vi "SavedSettingsItemData.vi"(8 "error in (no error)":errorcluster, 9 "Description":string, 10 "Title":string, 11 "CtrlTree in":refnum<vi>) -> (0 "error out":errorcluster, 2 "Is Empty":bool, 3 "Data to be saved":string[](array[string]))   [LabVIEW 2021]
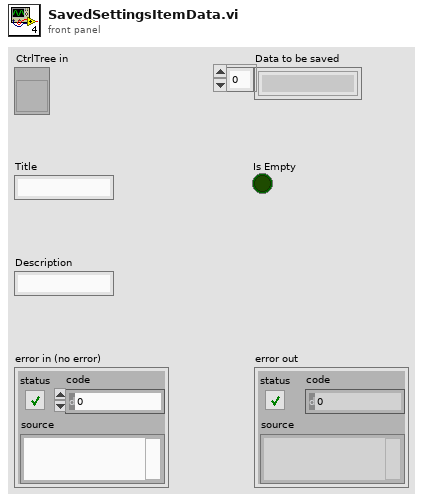
[diagram p1: front panel]
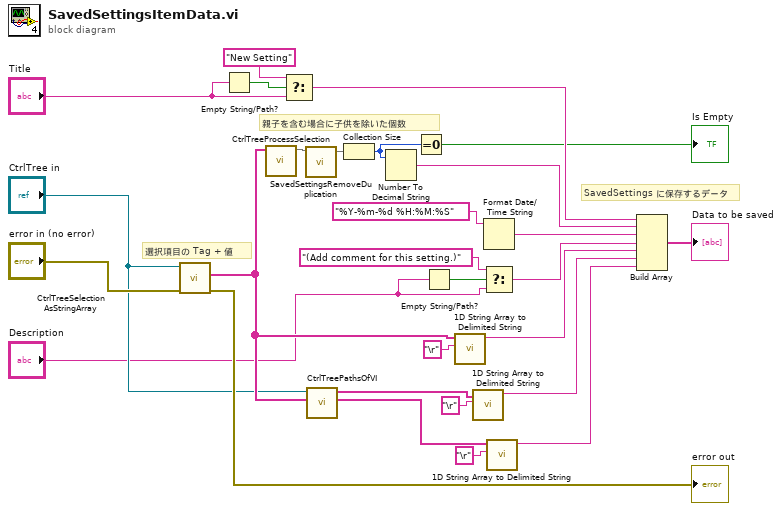
[diagram p0: block diagram]
diagram:
  # "親子を含む場合に子供を除いた個数"
  # "SavedSettings に保存するデータ"
  # "選択項目の Tag + 値"
  n1 = call "CtrlTreeSelectionAsStringArray.vi"("error in (no error)"="error in (no error)", "TreeControl in"="CtrlTree in") -> ("error out"=→"error out":errorcluster, "Selection"=w9:string[])  [unwired: 7 in, 1 out]
  n2 = Empty String/Path?(string/path="Title") -> (empty?=w24:bool)
  n3 = call "CtrlTreeProcessSelection.vi"("Selection"=w9) -> ("Map"=w10:map{string, string})  [unwired: 10 in]
  n4 = Select(t="New Setting" ("Left Cell String"), s=w24, f="Title") -> (s? t:f=w27:string)
  n5 = call "SavedSettingsRemoveDuplication.vi"("Saved Values"=w10) -> ("Saved Values (children removed)"=w12:map{string, string})  [unwired: 9 in, 1 out]
  n6 = call "CtrlTreePathsOfVI.vi"("Selection"=w9, "TreeControl in"="CtrlTree in") -> ("VI List"=w5:string[], "App List"=w3:string[])  [unwired: 8 in]
  n7 = Collection Size(1:w12) -> (0:w11:i32)
  n8 = Number To Decimal String(number=w11) -> (decimal integer string=w18:string)  [unwired: 1 in]
  n9 = Equal To 0?(x=w11) -> (x = 0?=→"Is Empty":bool)
  n10 = Empty String/Path?(string/path="Description") -> (empty?=w21:bool)
  n11 = call <vilib>:"1D String Array to Delimited String.vi"("delimiter"="\r", "string array"=w9) -> ("delimited string"=w20:string)  [unwired: 9 in]
  n12 = call <vilib>:"1D String Array to Delimited String.vi"("delimiter"="\r", "string array"=w3) -> ("delimited string"=w2:string)  [unwired: 9 in]
  n13 = Format Date/Time String(time format string (%c)="%Y-%m-%d %H:%M:%S") -> (date/time string=w17:string)  [unwired: 2 in]
  n14 = Select(t="(Add comment for this setting.)" ("element"), s=w21, f="Description") -> (s? t:f=w22:string)
  n15 = call <vilib>:"1D String Array to Delimited String.vi"("delimiter"="\r", "string array"=w5) -> ("delimited string"=w4:string)  [unwired: 9 in]
  n16 = Build Array(w27, w18, w17, w22, w20, w2, w4) -> (→"Data to be saved":string[])
